vi "dsdll_capture_wave_float32.vi"(8 "error in":errorcluster, 9 "transpose (false)":bool, 10 "samples count in":u32, 11 "dsdll instance in":T1={"dsdll path"=path "E:/LVprog/DirectSoundDLL/dsdll.dll", "dsdll handle"=[], "output devices"=[], "capture devices"=[]}) -> (0 "error out":errorcluster, 1 "int16 array":sgl[][](array[numeric]), 2 "samples count out":u32, 3 "dsdll instance out":T1, 4 "channels count":i32, 5 "time stamp [s]":dbl)   [LabVIEW 2018, in "dsdll.lvlib"]
doc: "Call this to capture waveform of specified length.\nThis VI si synchronous so it won't return untill entire waveform is recorded.\n\nOutput data format is 2D array of float32. Array organization:\n'transpose' = false: row = channels, columns = samples\n'transpose' = true: column = channels, rows = samples"
uses:
  dsdll.lvlib
  dsdll_instance.ctl
  dsdll_device_record.ctl
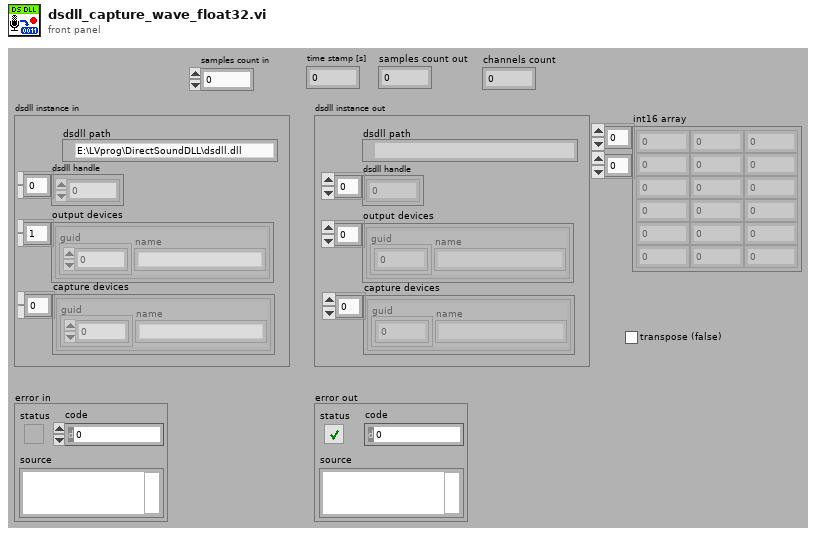
[diagram p1: front panel]
types:
  T1 = typedef "dsdll.lvlib/dsdll_instance.ctl" = cluster{"dsdll path":path, "dsdll handle":u8[], "output devices":T2[], "capture devices":T2[]}
  T2 = typedef "dsdll.lvlib/dsdll_device_record.ctl" = cluster{"guid":u8[], "name":string}
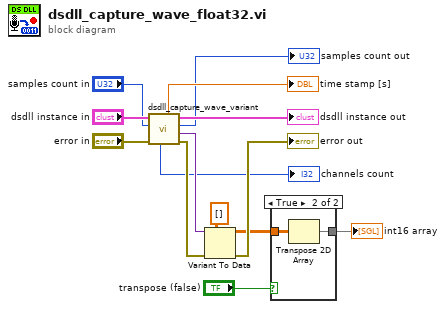
[diagram p0: block diagram]
diagram:
  n1 = call "dsdll_capture_wave_variant.vi"("error in"="error in", "samples count in"="samples count in", "dsdll instance in"="dsdll instance in") -> ("error out"=w6:errorcluster, "variant sample data"=w4:variant, "samples count out"=→"samples count out":u32, "dsdll instance out"=→"dsdll instance out":T1, "time stamp [s]"=→"time stamp [s]":dbl, "channels count"=→"channels count":u16)  [unwired: 2 in, 1 out]
  n2 = Variant To Data(error in=w6, type=sgl[][] [], Variant=w4) -> (data=w3:sgl[][], error out=→"error out":errorcluster)
  n3 = case shown="True" "transpose (false)" {
    tunnel: w3 -> [w15 w17]
    tunnel: [w15 w16] -> w9
    frame False {
    }
    frame True {
      n4 = Transpose 2D Array(2D array=w17) -> (transposed array=w16:sgl[][])
    }
  }
  "int16 array" <- w9
